vi "Get Default Impedance.vi"(8 "error in (no error)":errorcluster, 11 "VISA resource name":refnum<visa-resource-name>) -> (0 "error out":errorcluster, 2 "Default Impedance":i32, 3 "VISA resource name out":refnum<visa-resource-name>)   [LabVIEW 2011, in "Fluke 5XXX Series Multicalibrators.lvlib"]
doc: "This VI returns the power-up and reset default impedance used for dBm outputs (ac volts).\n\nNote:\n\nThis VI is available only for instrument model 5520A."
uses:
  Fluke 5XXX Series Multicalibrators.lvlib
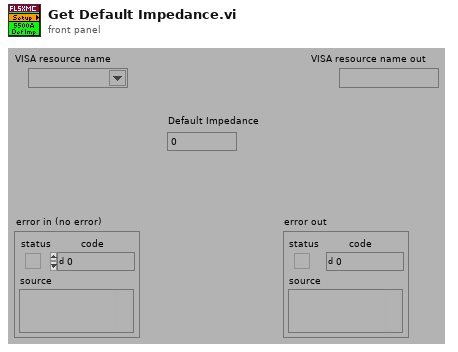
[diagram p1: front panel]
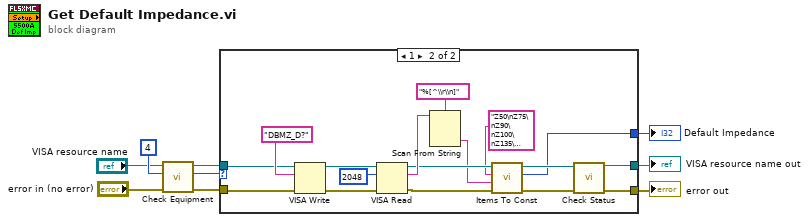
[diagram p0: block diagram]
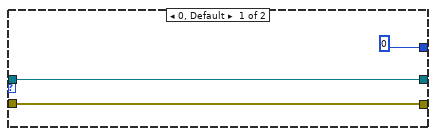
[diagram p2: hidden frame]
diagram:
  n1 = call "Check Equipment.vi"("error in (no error)"="error in (no error)", "Bit Mask"=4 ("Numeric"), "VISA resource name"="VISA resource name") -> ("error out"=w9:errorcluster, "Present?"=w8:u32, "VISA resource name out"=w7:refnum<visa-resource-name>)  [unwired: 6 in]
  n2 = case shown="1" w8 {
    tunnel: [w12 w23] -> w3
    tunnel: [w11 w22] -> w2
    tunnel: w9 -> [w12 w25]
    tunnel: w7 -> [w11 w24]
    tunnel: [0 w13] -> w1
    frame 0, Default {
    }
    frame 1 {
      n3 = VISA Write(VISA resource name=w24, write buffer="DBMZ_D?", error in (no error)=w25) -> (VISA resource name out=w28:refnum<visa-resource-name>, error out=w27:errorcluster)  [unwired: 1 out]
      n4 = VISA Read(VISA resource name=w28, byte count=u32 2048 ("byte count (0)"), error in (no error)=w27) -> (VISA resource name out=w19:refnum<visa-resource-name>, read buffer=w20:string, error out=w16:errorcluster)  [unwired: 1 out]
      n5 = Scan From String(format string="%[^\\r\\n]", input string=w20) -> (output 1=w14:string)  [unwired: 3 in, 3 out]
      n6 = call "Items To Const.vi"("error in (no error)"=w16, "String Item"=w14, "Multi-Line String"="Z50\nZ75\nZ90\nZ100\nZ135\nZ150\nZ300\nZ600\nZ900\nZ1000\nZ1200", "VISA resource name"=w19) -> ("error out"=w17:errorcluster, "Index"=w13:i32, "VISA resource name out"=w18:refnum<visa-resource-name>)  [unwired: 5 in]
      n7 = call "Check Status.vi"("VISA resource name"=w18, "error in (no error)"=w17) -> ("VISA resource name out"=w22:refnum<visa-resource-name>, "error out"=w23:errorcluster)  [unwired: 12 in]
    }
  }
  "Default Impedance" <- w1
  "VISA resource name out" <- w2
  "error out" <- w3
